vi "Robot.vi"(8 "Config":T1={"Gear Reduction"=15.0, "Wheel Radius (m)"=0.076, "# Motors"=1, "coeff of friction"=0.1, "Mass (kg)"=50.0, "Motor"={"Ke (V)"=0.0183, "R (ohms)"=0.09, "KT (Nm/A)"=0.0183, "Tf (Nm)"=0.4}}, 9 "WheelBase":dbl=30.0, 10 "Right Value":dbl=0.24600000000000002, 11 "Left Value":dbl=0.16228377222365817) -> (1 "Angle":dbl=2346.051245627821, 2 "Right Distance":dbl=829.590559330729, 3 "Left Distance":dbl=-398.79900037086566)   [LabVIEW 2019]
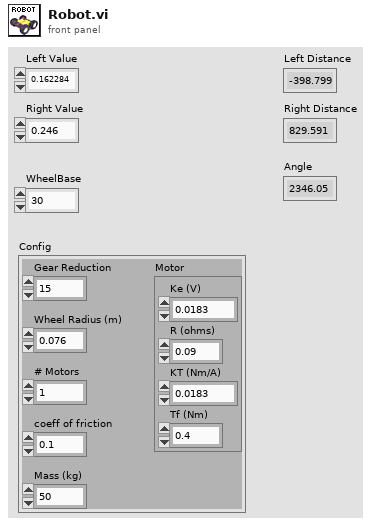
[diagram p1: front panel]
types:
  T1 = cluster{"Gear Reduction":dbl, "Wheel Radius (m)":dbl, "# Motors":u32, "coeff of friction":dbl, "Mass (kg)":dbl, "Motor":cluster{"Ke (V)":dbl, "R (ohms)":dbl, "KT (Nm/A)":dbl, "Tf (Nm)":dbl}}
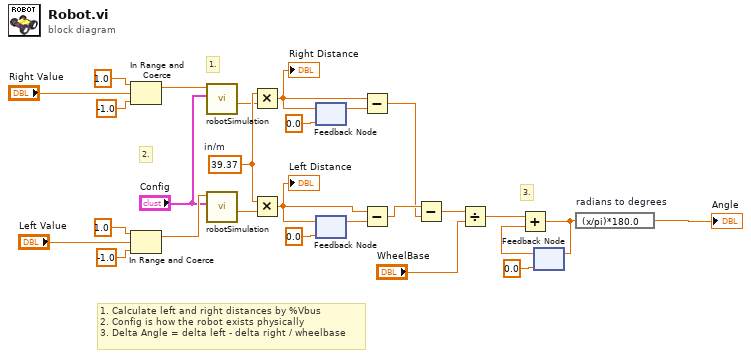
[diagram p0: block diagram]
diagram:
  w27 = 39.37  # in/m
  # "2."
  # "3."
  # "1."
  # "1. Calculate left and right distances by %Vbus\n2. Config is how the robot exists physically\n3. Delta Angle = delta left - delta right / wheelbase"
  n1 = In Range and Coerce(upper limit=1.0, x="Right Value", lower limit=-1.0) -> (coerced(x)=w7:dbl)  [unwired: 1 out]
  n2 = In Range and Coerce(upper limit=1.0, x="Left Value", lower limit=-1.0) -> (coerced(x)=w5:dbl)  [unwired: 1 out]
  n3 = call "robotSimulation.vi"("Config"="Config", "Duty Cycle"=w7) -> ("Position"=w6:dbl)  [unwired: 7 in, 2 out]
  n4 = call "robotSimulation.vi"("Config"="Config", "Duty Cycle"=w5) -> ("Position"=w3:dbl)  [unwired: 7 in, 2 out]
  n5 = Multiply(x=w27, y=w6) -> (x*y=w25:dbl)
  "Right Distance" <- w25
  n6 = Multiply(x=w27, y=w3) -> (x*y=w21:dbl)
  "Left Distance" <- w21
  n7 = feedback #1(0.0) -> (w26:dbl)
  n8 = feedback-in #1(w25) -> ()
  n9 = feedback #2(0.0) -> (w22:dbl)
  n10 = feedback-in #2(w21) -> ()
  n11 = Subtract(x=w25, y=w26) -> (x-y=w1:dbl)
  n12 = Subtract(x=w21, y=w22) -> (x-y=w2:dbl)
  n13 = Subtract(x=w2, y=w1) -> (x-y=w20:dbl)
  n14 = Divide(x=w20, y="WheelBase") -> (x/y=w18:dbl)
  n15 = feedback #3(0.0) -> (w17:dbl)
  n16 = Add(x=w18, y=w17) -> (x+y=w15:dbl)
  n17 = feedback-in #3(w15) -> ()
  n18 = expression code="(x/pi)*180.0" "radians to degrees"(w15) -> (→"Angle":dbl)
